vi "Set Serializer.vi"(8 "error in (no error)":errorcluster, 10 "Serializer":refnum<class "Serializer.lvclass">, 11 "Record in":refnum<class "Record.lvclass">) -> (0 "error out":errorcluster, 3 "Record out":refnum<class "Record.lvclass">)   [LabVIEW 2017, in "Error Log.lvlib" / "Record.lvclass"]
uses:
  Record.lvclass
  Serializer/Serializer.lvclass
  Record.lvclass/Record.ctl
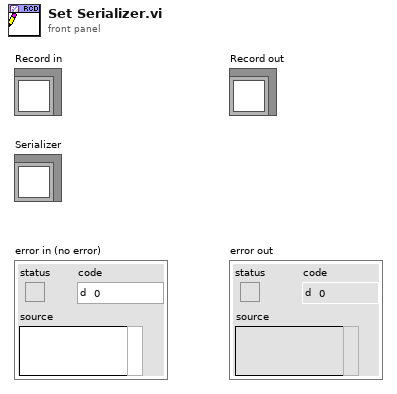
[diagram p1: front panel]
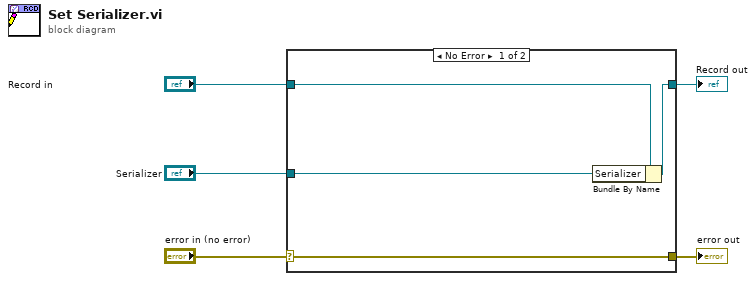
[diagram p0: block diagram]
diagram:
  n1 = case shown="No Error" "error in (no error)" {
    selector: "error in (no error)" -> [w9 w10]
    tunnel: [w9 w10] -> w4
    tunnel: [w7 w11] -> w2
    tunnel: "Record in" -> [w8 w11]
    tunnel: "Serializer" -> [w6 _]
    frame No Error {
      n2 = Bundle By Name(cluster=w8, "Serializer"=w6) -> (w7:refnum<class "Record.lvclass">)
    }
    frame Error {
    }
  }
  "error out" <- w4
  "Record out" <- w2
